vi "Get Board Info From Repo.vi"() -> (1 "Sorted ID":u32[](array[numeric]), 2 "Sorted Fam":u32[](array[numeric]), 3 "Sorted name":string[](array[string]))   [LabVIEW 2019, in "LINXx.lvlib"]
doc: "Get family/IDs from installed LINX library"
uses:
  LINXx.lvlib
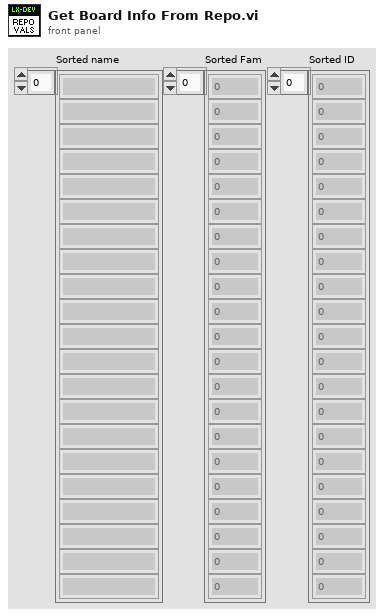
[diagram p1: front panel]
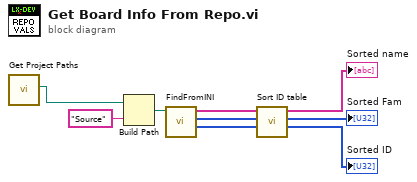
[diagram p0: block diagram]
diagram:
  n1 = call "Get Project Paths.vi"() -> ("Firmware path"=w1:path)  [unwired: 8 in, 3 out]
  n2 = Build Path(base path=w1, name or relative path="Source") -> (appended path=w8:path)
  n3 = call "FindFromINI.vi"("INI folder"=w8) -> ("IDs"=w2:u32[], "Families"=w3:u32[], "Names"=w4:string[])  [unwired: 7 in, 1 out]
  n4 = call "Sort ID table.vi"("ID"=w2, "Family"=w3, "Name"=w4) -> ("Sorted ID"=→"Sorted ID":u32[], "Sorted Fam"=→"Sorted Fam":u32[], "Sorted name"=→"Sorted name":string[])  [unwired: 6 in]
